vi "Curtin1_FavLists.vi"(6 "Task":enum16{"Save", "Read", "List", "Delete"}(ring), 8 "Default":string="favorites", 9 "List Name":string="favorites", 10 "description in":string, 11 "Files":T1[](array[typedef])) -> (1 "String":string, 2 "description out":string, 3 "Lists":string[](array[string]), 5 "Files Out":T1[](array[typedef]))   [LabVIEW 2022 SP3]
uses:
  Curtin1_Label.ctl
panel:
  out "error out":errorcluster
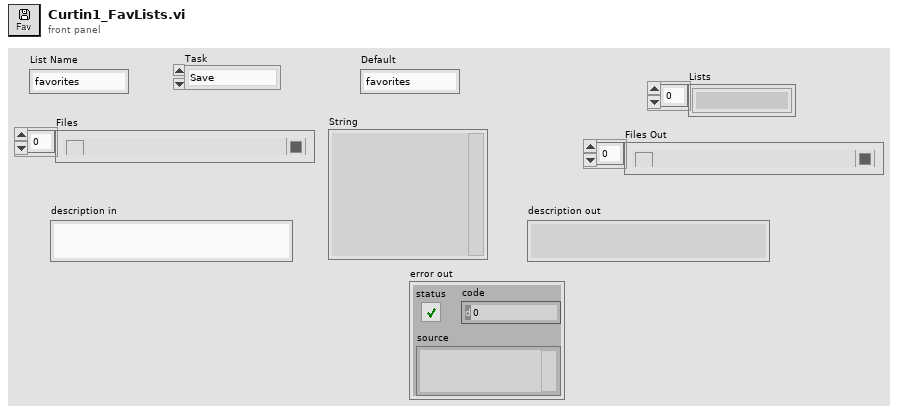
[diagram p1: front panel]
types:
  T1 = typedef "Curtin1_Label.ctl" = cluster{"Show?":bool, "Name":string, "Color":u32, "Path":path, "Show Notes":bool}
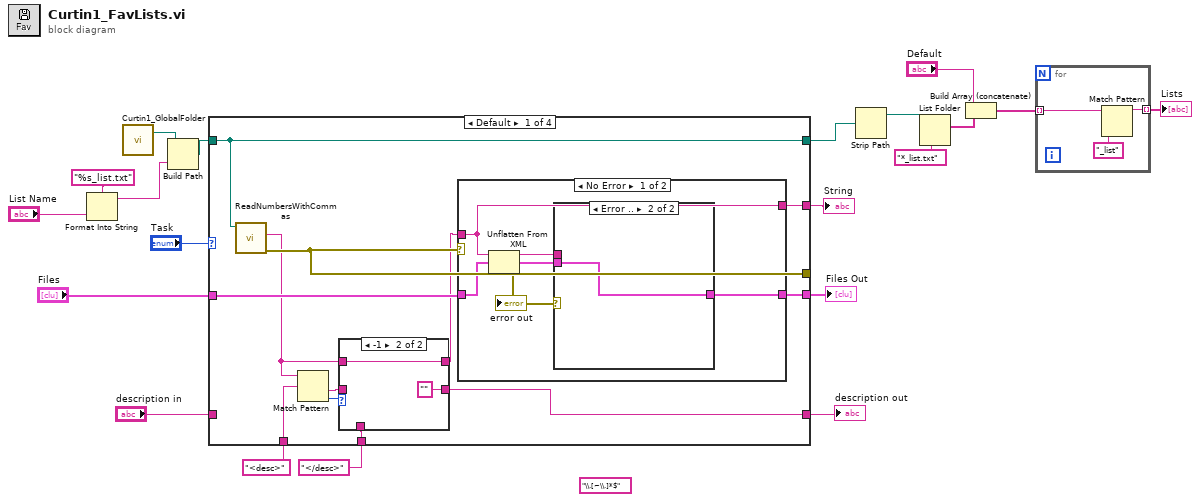
[diagram p0: block diagram]
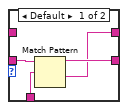
[diagram p2: hidden frame]
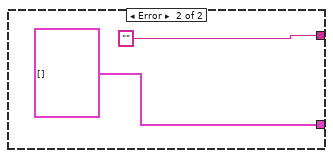
[diagram p4: hidden frame]
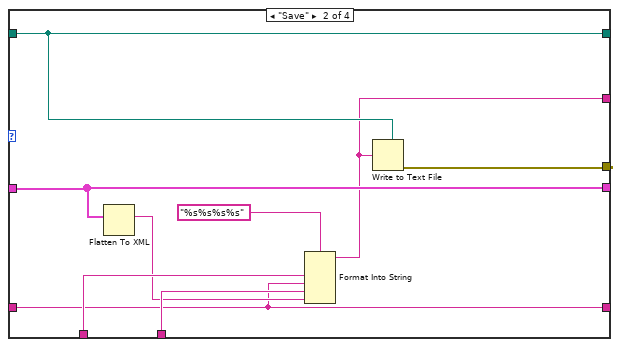
[diagram p5: hidden frame]
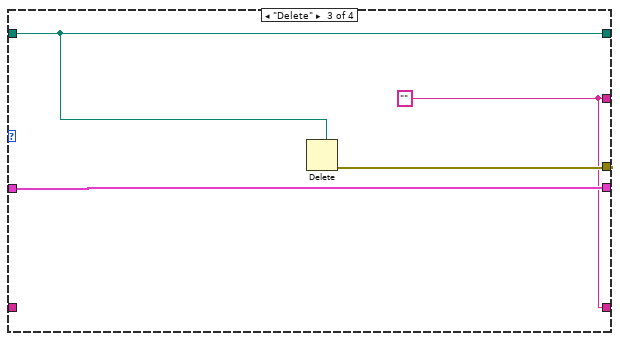
[diagram p6: hidden frame]
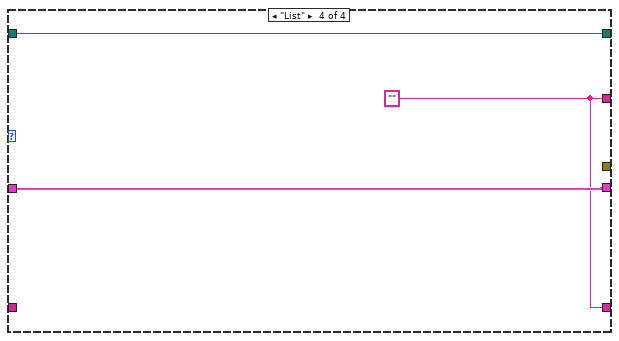
[diagram p7: hidden frame]
diagram:
  (unwired) "\\.[~\\.]*$" ("regular expression")
  n1 = Format Into String(format string="%s_list.txt" ("name or relative path"), "List Name") -> (resulting string=w16:string)  [unwired: 2 in, 1 out]
  n2 = call "Curtin1_GlobalFolder.vi"() -> ("LabVIEW Data Path"=w5:path)  [unwired: 1 in, 1 out]
  n3 = Build Path(base path=w5, name or relative path=w16) -> (appended path=w8:path)
  n4 = case shown="Default" "Task" {
    tunnel: "Files" -> [w31 w55 w59 w63]
    tunnel: [w29 w56 w60 _] -> _
    tunnel: [w32 w55 w59 w63] -> w14
    tunnel: [w30 w52 w57 w61] -> w18
    tunnel: [w22 w54 w58 w62] -> w7
    tunnel: w8 -> [w22 w54 w58 w62]
    tunnel: [w23 w48 w57 w61] -> w4
    tunnel: "description in" -> [_ w48 _ _]
    tunnel: "<desc>" ("regular expression") -> [w28 w51 _ _]
    tunnel: "</desc>" ("regular expression") -> [w24 w50 _ _]
    frame Default {
      n5 = call "ReadNumbersWithCommas.vi"("file (use dialog)"=w22) -> ("error out"=w29:errorcluster, "text"=w26:string)  [unwired: 7 in, 2 out]
      n6 = Match Pattern(string=w26, regular expression=w28) -> (after substring=w25:string, offset past match=w27:i32)  [unwired: 1 in, 2 out]
      n7 = case shown="-1" w27 {
        tunnel: [w33 w38] -> w21
        tunnel: w26 -> [_ w38]
        tunnel: w25 -> [w36 _]
        tunnel: w24 -> [w35 _]
        tunnel: [w34 "" ("text")] -> w23
        frame Default {
          n8 = Match Pattern(string=w36, regular expression=w35) -> (before substring=w34:string, after substring=w33:string)  [unwired: 1 in, 2 out]
        }
        frame -1 {
        }
      }
      n9 = case shown="No Error" w29 {
        tunnel: [w40 T1[] [] ("Files")] -> w32
        tunnel: w21 -> [w41 _]
        tunnel: w31 -> [w43 _]
        tunnel: [w41 ""] -> w30
        frame No Error {
          n10 = Unflatten From XML(xml string=w41, type=w43) -> (value=w39:T1[], error out=w42:errorcluster)  [unwired: 1 in]
          "error out" <- w42
          n11 = case shown="Error .." w42 {
            tunnel: w41 -> [_ _]
            tunnel: [w44 w45] -> w40
            tunnel: w39 -> [w44 w45]
            frame No Error {
            }
            frame Error {
            }
          }
        }
        frame Error {
        }
      }
    }
    frame "Save" {
      n12 = Flatten To XML(6:w55) -> (2:w49:string)
      n13 = Format Into String(format string="%s%s%s%s", w51, w48, w50, w49) -> (resulting string=w52:string)  [unwired: 2 in, 1 out]
      n14 = Write to Text File(file (use dialog)=w54, text=w52) -> (error out=w56:errorcluster)  [unwired: 2 in, 2 out]
    }
    frame "Delete" {
      w57 = "" ("spreadsheet string")
      n15 = Delete(path (use dialog)=w58) -> (error out=w60:errorcluster)  [unwired: 4 in, 2 out]
    }
    frame "List" {
      w61 = "" ("spreadsheet string")
    }
  }
  "String" <- w18
  "Files Out" <- w14
  "description out" <- w4
  n16 = Strip Path(path=w7) -> (stripped path=w13:path)  [unwired: 1 out]
  n17 = List Folder(path=w13, pattern="*_list.txt") -> (filenames=w11:string[])  [unwired: 2 in, 3 out]
  n18 = Build Array (concatenate)("Default", w11) -> (w12:string[])
  n19 = for {
    tunnel: [w65] -> w9 mode=indexing
    tunnel: w12 -> [w64] mode=indexing
    n20 = Match Pattern(string=w64, regular expression="_list") -> (before substring=w65:string)  [unwired: 4 out]
  }
  "Lists" <- w9
